vi "Read Dog.vi"(8 "error in (no error)":errorcluster, 11 "Dog Test in":refnum<class "Dog Test.lvclass">) -> (0 "error out":errorcluster, 2 "Dog.lvclass":refnum<class "Dog.lvclass">, 3 "Dog Test out":refnum<class "Dog Test.lvclass">)   [LabVIEW 2020, in "Dog Test.lvclass"]
doc: "Read Dog"
uses:
  Dog Test.lvclass
  C:/git/astemes-lunit-test-inheritance/builds/Test Inheritance/examples/astemes/LUnit Test Inheritance/Animal Test Classes/Animal Test/Animal Test.lvclass
  Animal Classes/Dog/Dog.lvclass
  Animal Test/Animal Test.lvclass
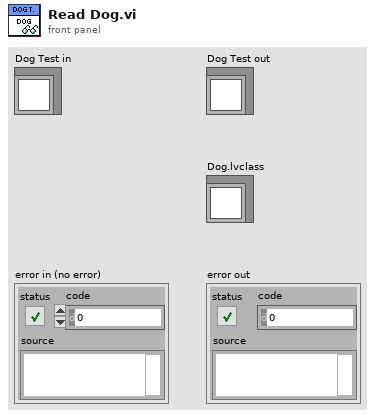
[diagram p1: front panel]
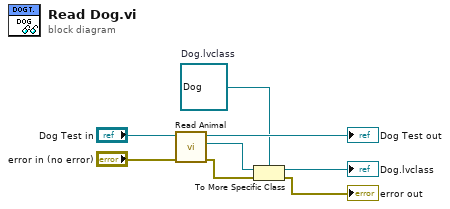
[diagram p0: block diagram]
diagram:
  w4 = refnum<class "Dog.lvclass"> refnum  # Dog.lvclass
  n1 = call "Read Animal.vi"("error in (no error)"="error in (no error)", "Animal Test In"="Dog Test in") -> ("error out"=w5:errorcluster, "Animal.lvclass"=w3:refnum<class "Animal.lvclass">, "Animal Test Out"=→"Dog Test out":refnum<class "Dog Test.lvclass">)  [unwired: 7 in]
  n2 = To More Specific Class(target class=w4, reference=w3, error in=w5) -> (specific class reference=→"Dog.lvclass":refnum<class "Dog.lvclass">, error out=→"error out":errorcluster)
